vi "Variant_UpdateClusterElements.vi"(7 "Cluster Name (ignored if cluster)":string, 9 "Element name":string, 10 "Element":variant, 11 "Cluster in":variant) -> (3 "Cluster out":variant)   [LabVIEW 2013]
uses:
  TypeDescriptor/TypeDescriptor_GetName.vi
  TypeDescriptor/TypeDescriptor_GetPString.vi
  TypeDescriptor/TypeDescriptor_SetName.vi
  OpenVariant.lvlib
  TypeDescriptor/OpenDescriptor.lvlib
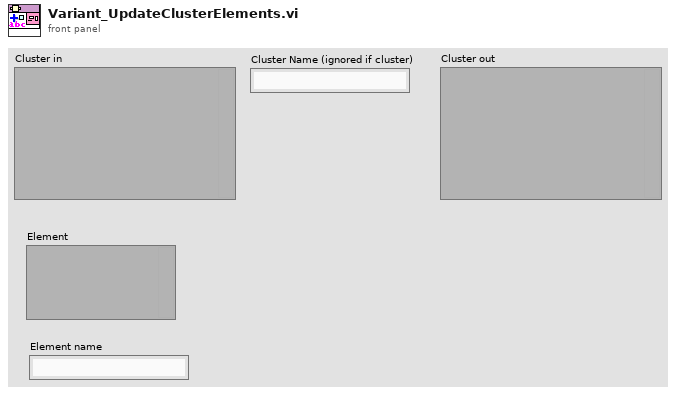
[diagram p1: front panel]
types:
  T1 = typedef "Type Descriptor I16 Array.ctl" = T2[]
  T2 = typedef "Type Descriptor I16.ctl" = i16
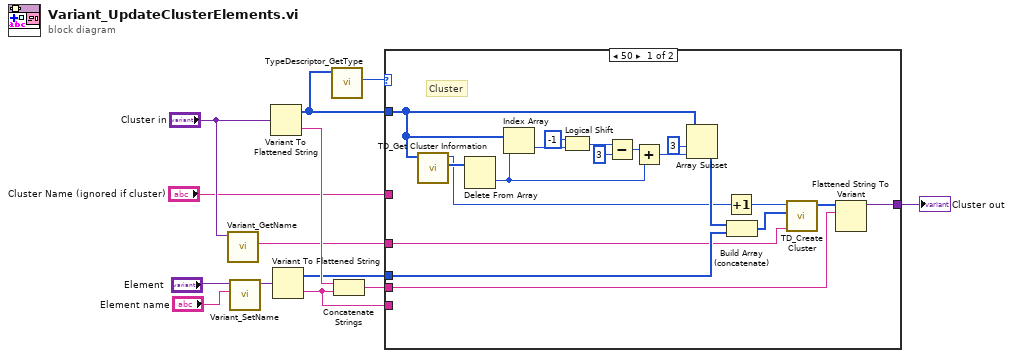
[diagram p0: block diagram]
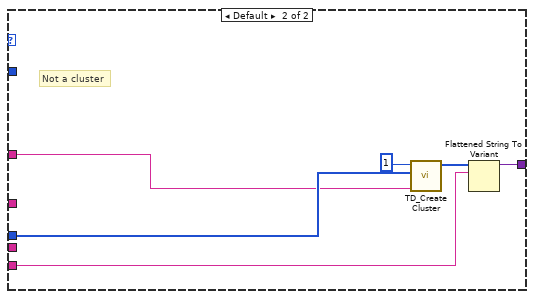
[diagram p2: hidden frame]
diagram:
  n1 = call "Variant_GetName.vi"("Variant"="Cluster in") -> ("Name"=w5:string)  [unwired: 8 in, 2 out]
  n2 = call "Variant_SetName.vi"("Name"="Element name", "Variant"="Element") -> ("Named Variant"=w9:variant)  [unwired: 9 in]
  n3 = Variant To Flattened String(Variant="Cluster in") -> (data string=w13:string, 1:w4:i16[])
  n4 = Variant To Flattened String(Variant=w9) -> (data string=w2:string, 1:w12:i16[])
  n5 = call "TypeDescriptor_GetType.vi"("type descriptor"=w4) -> ("Type"=w3:u8)  [unwired: 9 in, 1 out]
  n6 = Concatenate Strings(w13, w2) -> (w7:string)
  n7 = case shown="50" w3 {
    tunnel: w12 -> [w32 w35]
    tunnel: [w29 w37] -> w8
    tunnel: w7 -> [w28 _]
    tunnel: w5 -> [w19 _]
    tunnel: w4 -> [w14 _]
    tunnel: w2 -> [_ w34]
    tunnel: "Cluster Name (ignored if cluster)" -> [_ w33]
    frame 80 {
      # "Cluster"
      n8 = call <vilib>:"TD_Get Cluster Information.vi"("Type descriptor"=w14) -> ("Contained TD Offsets"=w25:i32[], "Number of Elements"=w18:i32)  [unwired: 9 in]
      n9 = Delete From Array(array=w25) -> (deleted portion=w17:i32)  [unwired: 2 in, 1 out]
      n10 = Index Array(array=w14, index=w17) -> (element=w23:i16)
      n11 = Logical Shift(y=i16 -1, x=w23) -> (x << y=w22:i16)
      n12 = Subtract(x=w22, y=3 ("index")) -> (x-y=w21:i32)
      n13 = Add(x=w21, y=w17) -> (x+y=w20:i32)
      n14 = Array Subset(array=w14, index=3, length=w20) -> (w26:i16[])
      n15 = Increment(x=w18) -> (x+1=w27:i32)
      n16 = Build Array (concatenate)(w26, w32) -> (w31:i16[])
      n17 = call <vilib>:"TD_Create Cluster.vi"("Name"=w19, "Concatenated Elts"=w31, "N Elts"=w27) -> ("ClusterTD"=w30:T1)  [unwired: 8 in]
      n18 = Flattened String To Variant(6:w28, 7:w30) -> (3:w29:variant)  [unwired: 1 in, 1 out]
    }
    frame Default {
      # "Not a cluster"
      n19 = call <vilib>:"TD_Create Cluster.vi"("Name"=w33, "Concatenated Elts"=w35, "N Elts"=1 ("x+1")) -> ("ClusterTD"=w38:T1)  [unwired: 8 in]
      n20 = Flattened String To Variant(6:w34, 7:w38) -> (3:w37:variant)  [unwired: 1 in, 1 out]
    }
  }
  "Cluster out" <- w8
